vi "Read Axis-parameters.vi"(8 "error in (no error)":errorcluster, 11 "DelayLine in":refnum<class "DelayLine.lvclass">) -> (0 "error out":errorcluster, 2 "Axis-parameters":T1(array[cluster]), 3 "DelayLine out":refnum<class "DelayLine.lvclass">)   [LabVIEW 2016, in "DelayLine.lvclass"]
uses:
  DelayLine.lvclass
  DelayLine.lvclass/DelayLine.ctl
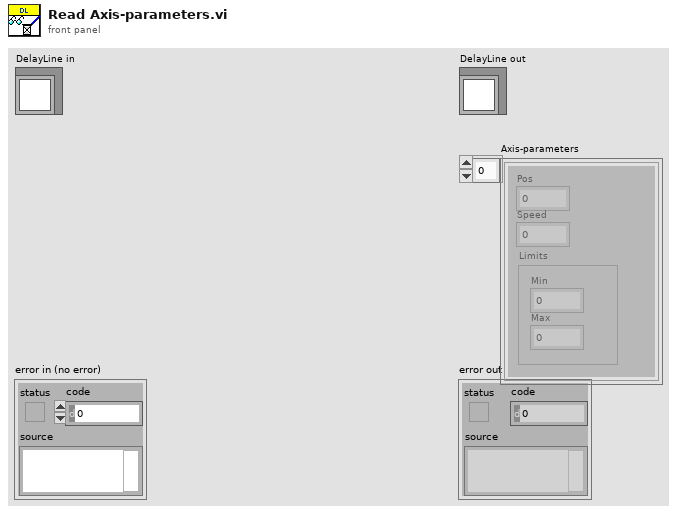
[diagram p1: front panel]
types:
  T1 = cluster{"Pos":dbl, "Speed":dbl, "Limits":cluster{"Min":dbl, "Max":dbl}}[]
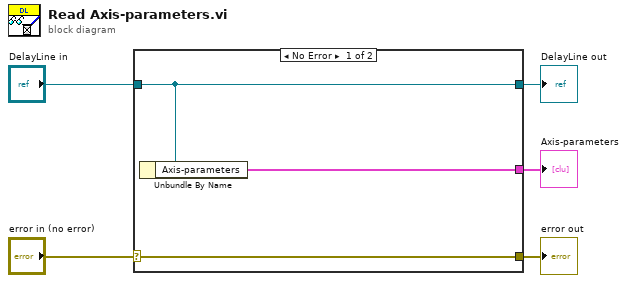
[diagram p0: block diagram]
diagram:
  n1 = case shown="No Error" "error in (no error)" {
    selector: "error in (no error)" -> [w8 w9]
    tunnel: [w8 w9] -> w4
    tunnel: [w7 w10] -> w2
    tunnel: "DelayLine in" -> [w7 w10]
    tunnel: [w6 _] -> w1
    frame No Error {
      n2 = Unbundle By Name(w7) -> ("Axis-parameters"=w6:T1)
    }
    frame Error {
    }
  }
  "error out" <- w4
  "DelayLine out" <- w2
  "Axis-parameters" <- w1
